vi "TCP Communicator - Active1.vi"() -> ()   [LabVIEW 2019]
panel:
  out "MC_Receive":T1 {"MirrorCoverControlScheme"."Time" format="%<%Y-%m-%d %H:%M:%S>T"; "MirrorCoverControllerConfig"."Time" format="%<%Y-%m-%d %H:%M:%S>T"; "MirrorCoverMotor-All"."MirrorCoverMotor-00"."Time" format="%<%Y-%m-%d %H:%M:%S>T"; "MirrorCoverMotor-All"."MirrorCoverMotor-01"."Time" format="%<%Y-%m-%d %H:%M:%S>T"; "MirrorCoverMotor-All"."MirrorCoverMotor-02"."Time" format="%<%Y-%m-%d %H:%M:%S>T"; "MirrorCoverMotor-All"."MirrorCoverMotor-03"."Time" format="%<%Y-%m-%d %H:%M:%S>T"; "MirrorCoverMotor-All"."MirrorCoverMotor-04"."Time" format="%<%Y-%m-%d %H:%M:%S>T"; "MirrorCoverMotor-All"."MirrorCoverMotor-05"."Time" format="%<%Y-%m-%d %H:%M:%S>T"; "MirrorCoverMotor-All"."MirrorCoverMotor-06"."Time" format="%<%Y-%m-%d %H:%M:%S>T"; "MirrorCoverMotor-All"."MirrorCoverMotor-07"."Time" format="%<%Y-%m-%d %H:%M:%S>T"}
  in  "stop":bool
  in  "MC_Send":T1 {"MirrorCoverControlScheme"."Time" format="%<%Y-%m-%d %H:%M:%S>T"; "MirrorCoverControllerConfig"."Time" format="%<%Y-%m-%d %H:%M:%S>T"; "MirrorCoverMotor-All"."MirrorCoverMotor-00"."Time" format="%<%Y-%m-%d %H:%M:%S>T"; "MirrorCoverMotor-All"."MirrorCoverMotor-01"."Time" format="%<%Y-%m-%d %H:%M:%S>T"; "MirrorCoverMotor-All"."MirrorCoverMotor-02"."Time" format="%<%Y-%m-%d %H:%M:%S>T"; "MirrorCoverMotor-All"."MirrorCoverMotor-03"."Time" format="%<%Y-%m-%d %H:%M:%S>T"; "MirrorCoverMotor-All"."MirrorCoverMotor-04"."Time" format="%<%Y-%m-%d %H:%M:%S>T"; "MirrorCoverMotor-All"."MirrorCoverMotor-05"."Time" format="%<%Y-%m-%d %H:%M:%S>T"; "MirrorCoverMotor-All"."MirrorCoverMotor-06"."Time" format="%<%Y-%m-%d %H:%M:%S>T"; "MirrorCoverMotor-All"."MirrorCoverMotor-07"."Time" format="%<%Y-%m-%d %H:%M:%S>T"}
  out "MC_Send 2":T1 {"MirrorCoverControlScheme"."Time" format="%<%Y-%m-%d %H:%M:%S>T"; "MirrorCoverControllerConfig"."Time" format="%<%Y-%m-%d %H:%M:%S>T"; "MirrorCoverMotor-All"."MirrorCoverMotor-00"."Time" format="%<%Y-%m-%d %H:%M:%S>T"; "MirrorCoverMotor-All"."MirrorCoverMotor-01"."Time" format="%<%Y-%m-%d %H:%M:%S>T"; "MirrorCoverMotor-All"."MirrorCoverMotor-02"."Time" format="%<%Y-%m-%d %H:%M:%S>T"; "MirrorCoverMotor-All"."MirrorCoverMotor-03"."Time" format="%<%Y-%m-%d %H:%M:%S>T"; "MirrorCoverMotor-All"."MirrorCoverMotor-04"."Time" format="%<%Y-%m-%d %H:%M:%S>T"; "MirrorCoverMotor-All"."MirrorCoverMotor-05"."Time" format="%<%Y-%m-%d %H:%M:%S>T"; "MirrorCoverMotor-All"."MirrorCoverMotor-06"."Time" format="%<%Y-%m-%d %H:%M:%S>T"; "MirrorCoverMotor-All"."MirrorCoverMotor-07"."Time" format="%<%Y-%m-%d %H:%M:%S>T"}
  in  "Port":u16=6342
  in  "Machine":string="192.168.150.83"
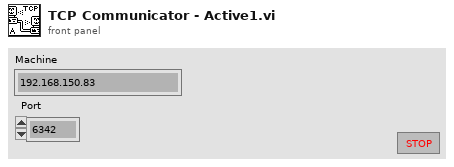
[diagram p1: front panel]
types:
  T1 = cluster{"MirrorCoverControlScheme":cluster{"Cold Start":bool, "Configuration":bool, "Start":bool, "Pointing/Tracking":bool, "Standby":bool, "Stop":bool, "Shutdown":bool, "Start Calibration":bool, "Start Maintenance":bool, "Status":i16, "Time ":timestamp}, "MirrorCoverControllerConfig":cluster{"ID":dbl, "K_P Config":dbl, "K_I Config":dbl, "K_D Config":dbl, "Status":i16, "Time ":timestamp}, "MirrorCoverMotor-All":cluster{"MirrorCoverMotor-00":cluster{"ID":i32, "Enable":bool, "Direction":bool, "Brake":bool, "Built-In Encoder":u64, "Motor Voltage FB":bool, "Motor Current FB":u64, "Brake Voltage FB":bool, "Brake Current FB":u64, "Up Limit Switch":bool, "Down Limit Switch":bool, "Up Limit Config":u64, "Down Limit Config":u64, "Motor Current Limit Config":u64, "Brake Current Limit Config":u64, "Status":i16, "Time ":timestamp}, "MirrorCoverMotor-01":cluster{"ID":i32, "Enable":bool, "Direction":bool, "Brake":bool, "Built-In Encoder":u64, "Motor Voltage FB":bool, "Motor Current FB":u64, "Brake Voltage FB":bool, "Brake Current FB":u64, "Up Limit Switch":bool, "Down Limit Switch":bool, "Up Limit Config":u64, "Down Limit Config":u64, "Motor Current Limit Config":u64, "Brake Current Limit Config":u64, "Status":i16, "Time ":timestamp}, "MirrorCoverMotor-02":cluster{"ID":i32, "Enable":bool, "Direction":bool, "Brake":bool, "Built-In Encoder":u64, "Motor Voltage FB":bool, "Motor Current FB":u64, "Brake Voltage FB":bool, "Brake Current FB":u64, "Up Limit Switch":bool, "Down Limit Switch":bool, "Up Limit Config":u64, "Down Limit Config":u64, "Motor Current Limit Config":u64, "Brake Current Limit Config":u64, "Status":i16, "Time ":timestamp}, "MirrorCoverMotor-03":cluster{"ID":i32, "Enable":bool, "Direction":bool, "Brake":bool, "Built-In Encoder":u64, "Motor Voltage FB":bool, "Motor Current FB":u64, "Brake Voltage FB":bool, "Brake Current FB":u64, "Up Limit Switch":bool, "Down Limit Switch":bool, "Up Limit Config":u64, "Down Limit Config":u64, "Motor Current Limit Config":u64, "Brake Current Limit Config":u64, "Status":i16, "Time ":timestamp}, "MirrorCoverMotor-04":cluster{"ID":i32, "Enable":bool, "Direction":bool, "Brake":bool, "Built-In Encoder":u64, "Motor Voltage FB":bool, "Motor Current FB":u64, "Brake Voltage FB":bool, "Brake Current FB":u64, "Up Limit Switch":bool, "Down Limit Switch":bool, "Up Limit Config":u64, "Down Limit Config":u64, "Motor Current Limit Config":u64, "Brake Current Limit Config":u64, "Status":i16, "Time ":timestamp}, "MirrorCoverMotor-05":cluster{"ID":i32, "Enable":bool, "Direction":bool, "Brake":bool, "Built-In Encoder":u64, "Motor Voltage FB":bool, "Motor Current FB":u64, "Brake Voltage FB":bool, "Brake Current FB":u64, "Up Limit Switch":bool, "Down Limit Switch":bool, "Up Limit Config":u64, "Down Limit Config":u64, "Motor Current Limit Config":u64, "Brake Current Limit Config":u64, "Status":i16, "Time ":timestamp}, "MirrorCoverMotor-06":cluster{"ID":i32, "Enable":bool, "Direction":bool, "Brake":bool, "Built-In Encoder":u64, "Motor Voltage FB":bool, "Motor Current FB":u64, "Brake Voltage FB":bool, "Brake Current FB":u64, "Up Limit Switch":bool, "Down Limit Switch":bool, "Up Limit Config":u64, "Down Limit Config":u64, "Motor Current Limit Config":u64, "Brake Current Limit Config":u64, "Status":i16, "Time ":timestamp}, "MirrorCoverMotor-07":cluster{"ID":i32, "Enable":bool, "Direction":bool, "Brake":bool, "Built-In Encoder":u64, "Motor Voltage FB":bool, "Motor Current FB":u64, "Brake Voltage FB":bool, "Brake Current FB":u64, "Up Limit Switch":bool, "Down Limit Switch":bool, "Up Limit Config":u64, "Down Limit Config":u64, "Motor Current Limit Config":u64, "Brake Current Limit Config":u64, "Status":i16, "Time ":timestamp}}}
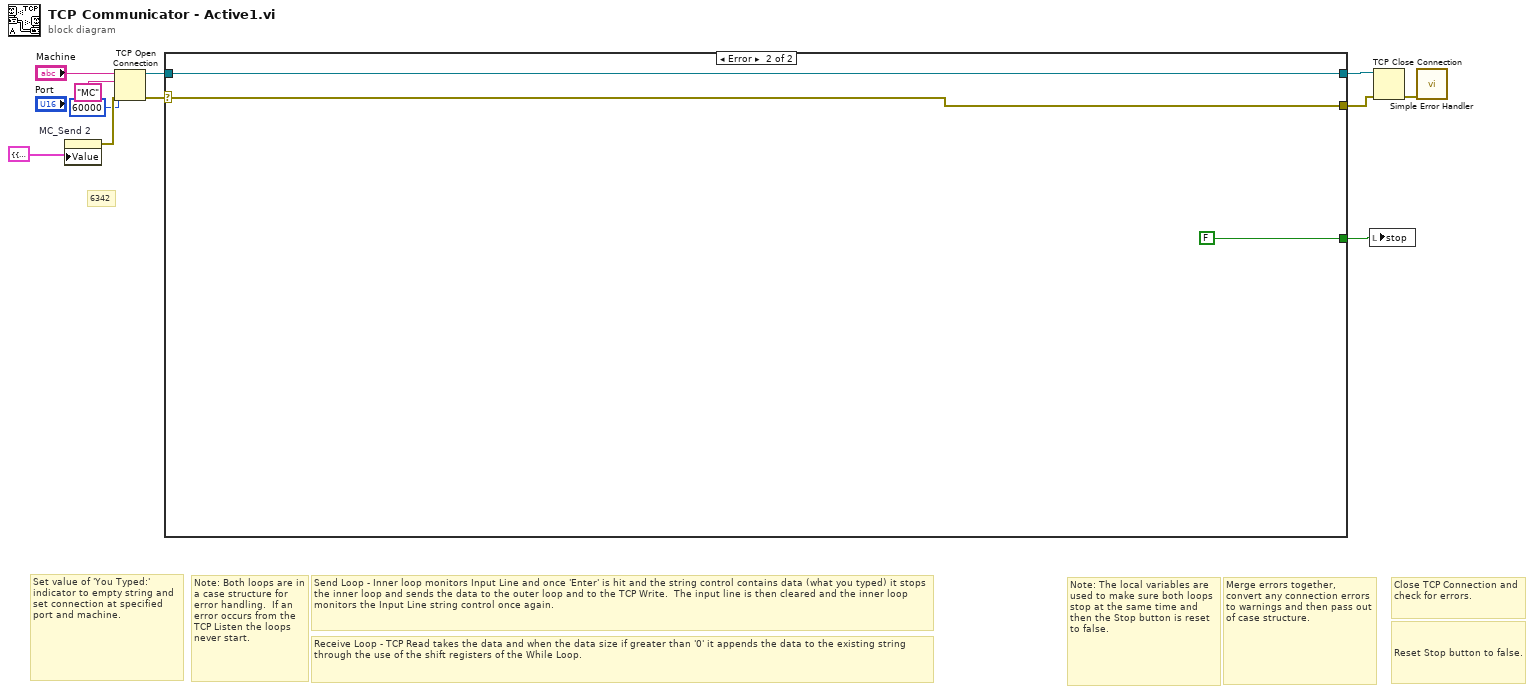
[diagram p0: block diagram]
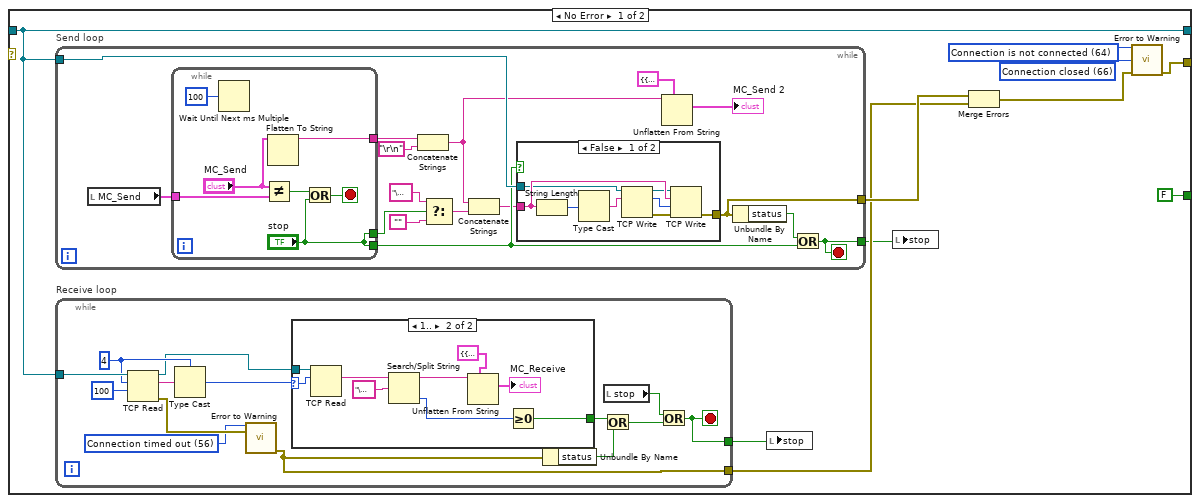
[diagram p2: hidden frame]
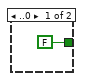
[diagram p3: hidden frame]
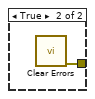
[diagram p4: hidden frame]
diagram:
  # "6342"
  # "Set value of 'You Typed:' indicator to empty string and set connection at specified port and machine."
  # "Send Loop - Inner loop monitors Input Line and once 'Enter' is hit and the string control contains data (what you typed) it stops the inner loop and sends the data to the outer loop and to the TCP Write.  The input line is then cleared and the inner loop monitors the Input Line string control once again."
  # "Receive Loop - TCP Read takes the data and when the data size if greater than '0' it appends the data to the existing string through the use of the shift registers of the While Loop."
  # "Note: The local variables are used to make sure both loops stop at the same time and then the Stop button is reset to false."
  # "Merge errors together, convert any connection errors to warnings and then pass out of case structure."
  # "Note: Both loops are in a case structure for error handling.  If an error occurs from the TCP Listen the loops never start."
  # "Close TCP Connection and check for errors."
  # "Reset Stop button to false."
  n1 = property on="MC_Send 2" class="Clust (strict)"("Value"=T1 {"MirrorCoverControlScheme"={"Cold Start"=FALSE, "Configuration"=FALSE, "Start"=FALSE, "Pointing/Tracking"=FALSE, "Standby"=FALSE, "Stop"=FALSE, "Shutdown"=FALSE, "Start Calibration"=FALSE, "Start Maintenance"=FALSE, "Status"=0, "Time "=timestamp(0 s since 1904-01-01)}, "MirrorCoverControllerConfig"={"ID"=0.0, "K_P Config"=0.0, "K_I Config"=0.0, "K_D Config"=0.0, "Status"=0, "Time "=timestamp(0 s since 1904-01-01)}, "MirrorCoverMotor-All"={"MirrorCoverMotor-00"={"ID"=0, "Enable"=FALSE, "Direction"=FALSE, "Brake"=FALSE, "Built-In Encoder"=0, "Motor Voltage FB"=FALSE, "Motor Current FB"=0, "Brake Voltage FB"=FALSE, "Brake Current FB"=0, "Up Limit Switch"=FALSE, "Down Limit Switch"=FALSE, "Up Limit Config"=0, "Down Limit Config"=0, "Motor Current Limit Config"=0, "Brake Current Limit Config"=0, "Status"=0, "Time "=timestamp(0 s since 1904-01-01)}, "MirrorCoverMotor-01"={"ID"=0, "Enable"=FALSE, "Direction"=FALSE, "Brake"=FALSE, "Built-In Encoder"=0, "Motor Voltage FB"=FALSE, "Motor Current FB"=0, "Brake Voltage FB"=FALSE, "Brake Current FB"=0, "Up Limit Switch"=FALSE, "Down Limit Switch"=FALSE, "Up Limit Config"=0, "Down Limit Config"=0, "Motor Current Limit Config"=0, "Brake Current Limit Config"=0, "Status"=0, "Time "=timestamp(0 s since 1904-01-01)}, "MirrorCoverMotor-02"={"ID"=0, "Enable"=FALSE, "Direction"=FALSE, "Brake"=FALSE, "Built-In Encoder"=0, "Motor Voltage FB"=FALSE, "Motor Current FB"=0, "Brake Voltage FB"=FALSE, "Brake Current FB"=0, "Up Limit Switch"=FALSE, "Down Limit Switch"=FALSE, "Up Limit Config"=0, "Down Limit Config"=0, "Motor Current Limit Config"=0, "Brake Current Limit Config"=0, "Status"=0, "Time "=timestamp(0 s since 1904-01-01)}, "MirrorCoverMotor-03"={"ID"=0, "Enable"=FALSE, "Direction"=FALSE, "Brake"=FALSE, "Built-In Encoder"=0, "Motor Voltage FB"=FALSE, "Motor Current FB"=0, "Brake Voltage FB"=FALSE, "Brake Current FB"=0, "Up Limit Switch"=FALSE, "Down Limit Switch"=FALSE, "Up Limit Config"=0, "Down Limit Config"=0, "Motor Current Limit Config"=0, "Brake Current Limit Config"=0, "Status"=0, "Time "=timestamp(0 s since 1904-01-01)}, "MirrorCoverMotor-04"={"ID"=0, "Enable"=FALSE, "Direction"=FALSE, "Brake"=FALSE, "Built-In Encoder"=0, "Motor Voltage FB"=FALSE, "Motor Current FB"=0, "Brake Voltage FB"=FALSE, "Brake Current FB"=0, "Up Limit Switch"=FALSE, "Down Limit Switch"=FALSE, "Up Limit Config"=0, "Down Limit Config"=0, "Motor Current Limit Config"=0, "Brake Current Limit Config"=0, "Status"=0, "Time "=timestamp(0 s since 1904-01-01)}, "MirrorCoverMotor-05"={"ID"=0, "Enable"=FALSE, "Direction"=FALSE, "Brake"=FALSE, "Built-In Encoder"=0, "Motor Voltage FB"=FALSE, "Motor Current FB"=0, "Brake Voltage FB"=FALSE, "Brake Current FB"=0, "Up Limit Switch"=FALSE, "Down Limit Switch"=FALSE, "Up Limit Config"=0, "Down Limit Config"=0, "Motor Current Limit Config"=0, "Brake Current Limit Config"=0, "Status"=0, "Time "=timestamp(0 s since 1904-01-01)}, "MirrorCoverMotor-06"={"ID"=0, "Enable"=FALSE, "Direction"=FALSE, "Brake"=FALSE, "Built-In Encoder"=0, "Motor Voltage FB"=FALSE, "Motor Current FB"=0, "Brake Voltage FB"=FALSE, "Brake Current FB"=0, "Up Limit Switch"=FALSE, "Down Limit Switch"=FALSE, "Up Limit Config"=0, "Down Limit Config"=0, "Motor Current Limit Config"=0, "Brake Current Limit Config"=0, "Status"=0, "Time "=timestamp(0 s since 1904-01-01)}, "MirrorCoverMotor-07"={"ID"=0, "Enable"=FALSE, "Direction"=FALSE, "Brake"=FALSE, "Built-In Encoder"=0, "Motor Voltage FB"=FALSE, "Motor Current FB"=0, "Brake Voltage FB"=FALSE, "Brake Current FB"=0, "Up Limit Switch"=FALSE, "Down Limit Switch"=FALSE, "Up Limit Config"=0, "Down Limit Config"=0, "Motor Current Limit Config"=0, "Brake Current Limit Config"=0, "Status"=0, "Time "=timestamp(0 s since 1904-01-01)}}} ("MC_Receive")) -> (error out=w3:errorcluster)  [unwired: 2 in, 1 out]
  n2 = TCP Open Connection(address="Machine", remote port or service name="MC" ("service name"), timeout ms (60000)=60000, error in (no error)=w3) -> (connection ID=w9:refnum<k5>, error out=w10:errorcluster)  [unwired: 1 in]
  n3 = case shown="Error" w10 {
    selector: w10 -> [_ w79]
    tunnel: [w18 w79] -> w7
    tunnel: w9 -> [w12 w80]
    tunnel: [w12 w80] -> w8
    tunnel: [FALSE FALSE] -> w5
    frame No Error {
      w19 = 66 items=["No Error", "Argument Error", "Memory Full", "Out of Zone", "End of File", "File Already Open", "Generic File IO Error", "File Not Found", "File Permission Error", "Disk Full", "Duplicate Path", "Too Many Files Open", "Not Enabled", "Resource File Not Found", "Cannot Add Resource", "Resource Not Found", "Image Not Found", "Image Memory Error", "Pen Does Not Exist", "Config Bad Type", "Config Token Not Found", "Config Parse Error", "Config Memory Error", "Bad External Code Format", "Bad External Code Offset", "External Code Not Present", "Null Window", "Destroy Window Mixup", "Null Menu", "Print Aborted", "Bad Print Record", "Print Driver Error", "Windows Error During Print", "Memory Error During Print", "Print Dialog Error", "Generic Print Error", "Invalid Device Refnum", "Device Not Found", "Device Parameter Error", "Device Unit Error", "Can't Open Device", "Device Call Aborted", "Generic Error", "Cancelled By User", "Object ID Too Low", "Object ID Too High", "Object Not In Heap", "Unknown Heap", "Bad DefProc ID", "DefProc Not In Table", "Message Out Of Range", "Null Method", "Unknown Message", "Manager Call Not Supported", "Bad address", "Connection In progress", "Connection timed out", "Connection is already in progress", "Network attribute not supported", "Network error", "Address in use", "System out of memory", "Connection aborted", "Connection refused", "Connection is not connected", "Connection is already connected", "Connection closed", "Initialize error (interapplication manager)", "Bad occurrence", "Wait on unbound occurrence handler", "Occurrence queue overflow", "Bad path", "Semaphore not signaled", "Unrecognized type (interapplication manager)"] ("3rd Error to Convert")
      w20 = 64 items=["No Error", "Argument Error", "Memory Full", "Out of Zone", "End of File", "File Already Open", "Generic File IO Error", "File Not Found", "File Permission Error", "Disk Full", "Duplicate Path", "Too Many Files Open", "Not Enabled", "Resource File Not Found", "Cannot Add Resource", "Resource Not Found", "Image Not Found", "Image Memory Error", "Pen Does Not Exist", "Config Bad Type", "Config Token Not Found", "Config Parse Error", "Config Memory Error", "Bad External Code Format", "Bad External Code Offset", "External Code Not Present", "Null Window", "Destroy Window Mixup", "Null Menu", "Print Aborted", "Bad Print Record", "Print Driver Error", "Windows Error During Print", "Memory Error During Print", "Print Dialog Error", "Generic Print Error", "Invalid Device Refnum", "Device Not Found", "Device Parameter Error", "Device Unit Error", "Can't Open Device", "Device Call Aborted", "Generic Error", "Cancelled By User", "Object ID Too Low", "Object ID Too High", "Object Not In Heap", "Unknown Heap", "Bad DefProc ID", "DefProc Not In Table", "Message Out Of Range", "Null Method", "Unknown Message", "Manager Call Not Supported", "Bad address", "Connection In progress", "Connection timed out", "Connection is already in progress", "Network attribute not supported", "Network error", "Address in use", "System out of memory", "Connection aborted", "Connection refused", "Connection is not connected", "Connection is already connected", "Connection closed", "Initialize error (interapplication manager)", "Bad occurrence", "Wait on unbound occurrence handler", "Occurrence queue overflow", "Bad path", "Semaphore not signaled", "Unrecognized type (interapplication manager)"] ("1st Error to Convert")
      n4 = while "Send loop" {
        tunnel: w12 -> [w60]
        tunnel: [w61] -> w13
        tunnel: [w56] -> w16
        stop <- w61 stop-if-true
        n5 = local read "MC_Send"() -> (w53:T1)
        n6 = while {
          tunnel: ["stop"] -> w58
          tunnel: ["stop"] -> w54
          tunnel: [w62] -> w49
          tunnel: w53 -> [w65]
          stop <- w66 stop-if-true
          n7 = Wait Until Next ms Multiple(millisecond multiple=u32 100) -> ()  [unwired: 1 out]
          n8 = Not Equal?(x="MC_Send", y=w65) -> (x != y?=w67:bool)
          n9 = Flatten To String(anything="MC_Send") -> (data string=w62:string)  [unwired: 3 in, 2 out]
          n10 = Or(x=w67, y="stop") -> (x .or. y?=w66:bool)
        }
        n11 = Concatenate Strings(w49, "\r\n") -> (w48:string)
        n12 = Select(t="\u0004", s=w58, f="") -> (s? t:f=w47:string)
        n13 = Concatenate Strings(w48, w47) -> (w46:string)
        n14 = case shown="False" w54 {
          tunnel: w46 -> [w73 _]
          tunnel: [w76 w77] -> w56
          tunnel: w60 -> [w70 _]
          frame False {
            n15 = String Length(string=w73) -> (length=w72:i32)
            n16 = Type Cast(x=w72) -> (*(type *) &x=w71:string)  [unwired: 1 in]
            n17 = TCP Write(connection ID=w70, data in=w71) -> (connection ID out=w69:refnum<k5>, bytes written=w74:i32, error out=w75:errorcluster)  [unwired: 2 in]
            n18 = TCP Write(connection ID=w69, data in=w73, error in (no error)=w75, 9:w74) -> (error out=w76:errorcluster)  [unwired: 2 out]
          }
          frame True {
            n19 = call <vilib>:"Clear Errors.vi"() -> ("error out"=w77:errorcluster)  [unwired: 6 in, 1 out]
          }
        }
        n20 = Unflatten From String(type=T1 {"MirrorCoverControlScheme"={"Cold Start"=FALSE, "Configuration"=FALSE, "Start"=FALSE, "Pointing/Tracking"=FALSE, "Standby"=FALSE, "Stop"=FALSE, "Shutdown"=FALSE, "Start Calibration"=FALSE, "Start Maintenance"=FALSE, "Status"=0, "Time "=timestamp(0 s since 1904-01-01)}, "MirrorCoverControllerConfig"={"ID"=0.0, "K_P Config"=0.0, "K_I Config"=0.0, "K_D Config"=0.0, "Status"=0, "Time "=timestamp(0 s since 1904-01-01)}, "MirrorCoverMotor-All"={"MirrorCoverMotor-00"={"ID"=0, "Enable"=FALSE, "Direction"=FALSE, "Brake"=FALSE, "Built-In Encoder"=0, "Motor Voltage FB"=FALSE, "Motor Current FB"=0, "Brake Voltage FB"=FALSE, "Brake Current FB"=0, "Up Limit Switch"=FALSE, "Down Limit Switch"=FALSE, "Up Limit Config"=0, "Down Limit Config"=0, "Motor Current Limit Config"=0, "Brake Current Limit Config"=0, "Status"=0, "Time "=timestamp(0 s since 1904-01-01)}, "MirrorCoverMotor-01"={"ID"=0, "Enable"=FALSE, "Direction"=FALSE, "Brake"=FALSE, "Built-In Encoder"=0, "Motor Voltage FB"=FALSE, "Motor Current FB"=0, "Brake Voltage FB"=FALSE, "Brake Current FB"=0, "Up Limit Switch"=FALSE, "Down Limit Switch"=FALSE, "Up Limit Config"=0, "Down Limit Config"=0, "Motor Current Limit Config"=0, "Brake Current Limit Config"=0, "Status"=0, "Time "=timestamp(0 s since 1904-01-01)}, "MirrorCoverMotor-02"={"ID"=0, "Enable"=FALSE, "Direction"=FALSE, "Brake"=FALSE, "Built-In Encoder"=0, "Motor Voltage FB"=FALSE, "Motor Current FB"=0, "Brake Voltage FB"=FALSE, "Brake Current FB"=0, "Up Limit Switch"=FALSE, "Down Limit Switch"=FALSE, "Up Limit Config"=0, "Down Limit Config"=0, "Motor Current Limit Config"=0, "Brake Current Limit Config"=0, "Status"=0, "Time "=timestamp(0 s since 1904-01-01)}, "MirrorCoverMotor-03"={"ID"=0, "Enable"=FALSE, "Direction"=FALSE, "Brake"=FALSE, "Built-In Encoder"=0, "Motor Voltage FB"=FALSE, "Motor Current FB"=0, "Brake Voltage FB"=FALSE, "Brake Current FB"=0, "Up Limit Switch"=FALSE, "Down Limit Switch"=FALSE, "Up Limit Config"=0, "Down Limit Config"=0, "Motor Current Limit Config"=0, "Brake Current Limit Config"=0, "Status"=0, "Time "=timestamp(0 s since 1904-01-01)}, "MirrorCoverMotor-04"={"ID"=0, "Enable"=FALSE, "Direction"=FALSE, "Brake"=FALSE, "Built-In Encoder"=0, "Motor Voltage FB"=FALSE, "Motor Current FB"=0, "Brake Voltage FB"=FALSE, "Brake Current FB"=0, "Up Limit Switch"=FALSE, "Down Limit Switch"=FALSE, "Up Limit Config"=0, "Down Limit Config"=0, "Motor Current Limit Config"=0, "Brake Current Limit Config"=0, "Status"=0, "Time "=timestamp(0 s since 1904-01-01)}, "MirrorCoverMotor-05"={"ID"=0, "Enable"=FALSE, "Direction"=FALSE, "Brake"=FALSE, "Built-In Encoder"=0, "Motor Voltage FB"=FALSE, "Motor Current FB"=0, "Brake Voltage FB"=FALSE, "Brake Current FB"=0, "Up Limit Switch"=FALSE, "Down Limit Switch"=FALSE, "Up Limit Config"=0, "Down Limit Config"=0, "Motor Current Limit Config"=0, "Brake Current Limit Config"=0, "Status"=0, "Time "=timestamp(0 s since 1904-01-01)}, "MirrorCoverMotor-06"={"ID"=0, "Enable"=FALSE, "Direction"=FALSE, "Brake"=FALSE, "Built-In Encoder"=0, "Motor Voltage FB"=FALSE, "Motor Current FB"=0, "Brake Voltage FB"=FALSE, "Brake Current FB"=0, "Up Limit Switch"=FALSE, "Down Limit Switch"=FALSE, "Up Limit Config"=0, "Down Limit Config"=0, "Motor Current Limit Config"=0, "Brake Current Limit Config"=0, "Status"=0, "Time "=timestamp(0 s since 1904-01-01)}, "MirrorCoverMotor-07"={"ID"=0, "Enable"=FALSE, "Direction"=FALSE, "Brake"=FALSE, "Built-In Encoder"=0, "Motor Voltage FB"=FALSE, "Motor Current FB"=0, "Brake Voltage FB"=FALSE, "Brake Current FB"=0, "Up Limit Switch"=FALSE, "Down Limit Switch"=FALSE, "Up Limit Config"=0, "Down Limit Config"=0, "Motor Current Limit Config"=0, "Brake Current Limit Config"=0, "Status"=0, "Time "=timestamp(0 s since 1904-01-01)}}} ("MC_Receive"), binary string=w48) -> (value=→"MC_Send 2":T1)  [unwired: 3 in, 2 out]
        n21 = Unbundle By Name(w56) -> ("status"=w55:bool)
        n22 = Or(x=w55, y=w54) -> (x .or. y?=w61:bool)
      }
      n23 = while "Receive loop" {
        tunnel: [w34] -> w15
        tunnel: [w29] -> w14
        tunnel: w12 -> [w35]
        stop <- w34 stop-if-true
        w24 = 4
        w30 = 56 items=["No Error", "Argument Error", "Memory Full", "Out of Zone", "End of File", "File Already Open", "Generic File IO Error", "File Not Found", "File Permission Error", "Disk Full", "Duplicate Path", "Too Many Files Open", "Not Enabled", "Resource File Not Found", "Cannot Add Resource", "Resource Not Found", "Image Not Found", "Image Memory Error", "Pen Does Not Exist", "Config Bad Type", "Config Token Not Found", "Config Parse Error", "Config Memory Error", "Bad External Code Format", "Bad External Code Offset", "External Code Not Present", "Null Window", "Destroy Window Mixup", "Null Menu", "Print Aborted", "Bad Print Record", "Print Driver Error", "Windows Error During Print", "Memory Error During Print", "Print Dialog Error", "Generic Print Error", "Invalid Device Refnum", "Device Not Found", "Device Parameter Error", "Device Unit Error", "Can't Open Device", "Device Call Aborted", "Generic Error", "Cancelled By User", "Object ID Too Low", "Object ID Too High", "Object Not In Heap", "Unknown Heap", "Bad DefProc ID", "DefProc Not In Table", "Message Out Of Range", "Null Method", "Unknown Message", "Manager Call Not Supported", "Bad address", "Connection In progress", "Connection timed out", "Connection is already in progress", "Network attribute not supported", "Network error", "Address in use", "System out of memory", "Connection aborted", "Connection refused", "Connection is not connected", "Connection is already connected", "Connection closed", "Initialize error (interapplication manager)", "Bad occurrence", "Wait on unbound occurrence handler", "Occurrence queue overflow", "Bad path", "Semaphore not signaled", "Unrecognized type (interapplication manager)"] ("1st Error to Convert")
        n24 = TCP Read(connection ID=w35, bytes to read=w24, 9:100) -> (connection ID out=w22:refnum<k5>, data out=w25:string, error out=w31:errorcluster)  [unwired: 2 in]
        n25 = Type Cast(type=w24, x=w25) -> (*(type *) &x=w23:i32)
        n26 = call <vilib>:"Error to Warning.vi"("1st Error to Convert"=w30, "error in"=w31) -> ("warning out"=w29:errorcluster)  [unwired: 13 in]
        n27 = case shown="1.." w23 {
          selector: w23 -> [_ w45]
          tunnel: [FALSE w40] -> w33
          tunnel: w22 -> [_ w44]
          frame ..0 {
          }
          frame 1.. {
            n28 = TCP Read(connection ID=w44, bytes to read=w45) -> (data out=w39:string)  [unwired: 3 in, 2 out]
            n29 = Search/Split String(string=w39, search string/char (-)="\u0004") -> (substring before match=w38:string, offset of match=w42:i32)  [unwired: 1 in, 1 out]
            n30 = Unflatten From String(type=T1 {"MirrorCoverControlScheme"={"Cold Start"=FALSE, "Configuration"=FALSE, "Start"=FALSE, "Pointing/Tracking"=FALSE, "Standby"=FALSE, "Stop"=FALSE, "Shutdown"=FALSE, "Start Calibration"=FALSE, "Start Maintenance"=FALSE, "Status"=0, "Time "=timestamp(0 s since 1904-01-01)}, "MirrorCoverControllerConfig"={"ID"=0.0, "K_P Config"=0.0, "K_I Config"=0.0, "K_D Config"=0.0, "Status"=0, "Time "=timestamp(0 s since 1904-01-01)}, "MirrorCoverMotor-All"={"MirrorCoverMotor-00"={"ID"=0, "Enable"=FALSE, "Direction"=FALSE, "Brake"=FALSE, "Built-In Encoder"=0, "Motor Voltage FB"=FALSE, "Motor Current FB"=0, "Brake Voltage FB"=FALSE, "Brake Current FB"=0, "Up Limit Switch"=FALSE, "Down Limit Switch"=FALSE, "Up Limit Config"=0, "Down Limit Config"=0, "Motor Current Limit Config"=0, "Brake Current Limit Config"=0, "Status"=0, "Time "=timestamp(0 s since 1904-01-01)}, "MirrorCoverMotor-01"={"ID"=0, "Enable"=FALSE, "Direction"=FALSE, "Brake"=FALSE, "Built-In Encoder"=0, "Motor Voltage FB"=FALSE, "Motor Current FB"=0, "Brake Voltage FB"=FALSE, "Brake Current FB"=0, "Up Limit Switch"=FALSE, "Down Limit Switch"=FALSE, "Up Limit Config"=0, "Down Limit Config"=0, "Motor Current Limit Config"=0, "Brake Current Limit Config"=0, "Status"=0, "Time "=timestamp(0 s since 1904-01-01)}, "MirrorCoverMotor-02"={"ID"=0, "Enable"=FALSE, "Direction"=FALSE, "Brake"=FALSE, "Built-In Encoder"=0, "Motor Voltage FB"=FALSE, "Motor Current FB"=0, "Brake Voltage FB"=FALSE, "Brake Current FB"=0, "Up Limit Switch"=FALSE, "Down Limit Switch"=FALSE, "Up Limit Config"=0, "Down Limit Config"=0, "Motor Current Limit Config"=0, "Brake Current Limit Config"=0, "Status"=0, "Time "=timestamp(0 s since 1904-01-01)}, "MirrorCoverMotor-03"={"ID"=0, "Enable"=FALSE, "Direction"=FALSE, "Brake"=FALSE, "Built-In Encoder"=0, "Motor Voltage FB"=FALSE, "Motor Current FB"=0, "Brake Voltage FB"=FALSE, "Brake Current FB"=0, "Up Limit Switch"=FALSE, "Down Limit Switch"=FALSE, "Up Limit Config"=0, "Down Limit Config"=0, "Motor Current Limit Config"=0, "Brake Current Limit Config"=0, "Status"=0, "Time "=timestamp(0 s since 1904-01-01)}, "MirrorCoverMotor-04"={"ID"=0, "Enable"=FALSE, "Direction"=FALSE, "Brake"=FALSE, "Built-In Encoder"=0, "Motor Voltage FB"=FALSE, "Motor Current FB"=0, "Brake Voltage FB"=FALSE, "Brake Current FB"=0, "Up Limit Switch"=FALSE, "Down Limit Switch"=FALSE, "Up Limit Config"=0, "Down Limit Config"=0, "Motor Current Limit Config"=0, "Brake Current Limit Config"=0, "Status"=0, "Time "=timestamp(0 s since 1904-01-01)}, "MirrorCoverMotor-05"={"ID"=0, "Enable"=FALSE, "Direction"=FALSE, "Brake"=FALSE, "Built-In Encoder"=0, "Motor Voltage FB"=FALSE, "Motor Current FB"=0, "Brake Voltage FB"=FALSE, "Brake Current FB"=0, "Up Limit Switch"=FALSE, "Down Limit Switch"=FALSE, "Up Limit Config"=0, "Down Limit Config"=0, "Motor Current Limit Config"=0, "Brake Current Limit Config"=0, "Status"=0, "Time "=timestamp(0 s since 1904-01-01)}, "MirrorCoverMotor-06"={"ID"=0, "Enable"=FALSE, "Direction"=FALSE, "Brake"=FALSE, "Built-In Encoder"=0, "Motor Voltage FB"=FALSE, "Motor Current FB"=0, "Brake Voltage FB"=FALSE, "Brake Current FB"=0, "Up Limit Switch"=FALSE, "Down Limit Switch"=FALSE, "Up Limit Config"=0, "Down Limit Config"=0, "Motor Current Limit Config"=0, "Brake Current Limit Config"=0, "Status"=0, "Time "=timestamp(0 s since 1904-01-01)}, "MirrorCoverMotor-07"={"ID"=0, "Enable"=FALSE, "Direction"=FALSE, "Brake"=FALSE, "Built-In Encoder"=0, "Motor Voltage FB"=FALSE, "Motor Current FB"=0, "Brake Voltage FB"=FALSE, "Brake Current FB"=0, "Up Limit Switch"=FALSE, "Down Limit Switch"=FALSE, "Up Limit Config"=0, "Down Limit Config"=0, "Motor Current Limit Config"=0, "Brake Current Limit Config"=0, "Status"=0, "Time "=timestamp(0 s since 1904-01-01)}}} ("MC_Receive"), binary string=w38) -> (value=→"MC_Receive":T1)  [unwired: 3 in, 2 out]
            n31 = Greater Or Equal To 0?(x=w42) -> (x >= 0?=w40:bool)
          }
        }
        n32 = Unbundle By Name(w29) -> ("status"=w28:bool)
        n33 = Or(x=w33, y=w28) -> (x .or. y?=w26:bool)
        n34 = local read "stop"() -> (w27:bool)
        n35 = Or(x=w27, y=w26) -> (x .or. y?=w34:bool)
      }
      n36 = local write "stop"(w15) -> ()
      n37 = local write "stop"(w13) -> ()
      n38 = Merge Errors(w16, w14) -> (w21:errorcluster)
      n39 = call <vilib>:"Error to Warning.vi"("1st Error to Convert"=w20, "3rd Error to Convert"=w19, "error in"=w21) -> ("warning out"=w18:errorcluster)  [unwired: 12 in]
    }
    frame Error {
    }
  }
  n40 = local write "stop"(w5) -> ()
  n41 = TCP Close Connection(connection ID=w8, error in (no error)=w7) -> (error out=w6:errorcluster)  [unwired: 1 in, 1 out]
  n42 = call <vilib>:"Simple Error Handler.vi"("error in (no error)"=w6) -> ()  [unwired: 4 in, 5 out]
